vi "Login副本.vi"() -> ()   [LabVIEW 2015]
uses:
  <userlib>/QMH/Message Queue/Support/Enqueue Message (Single).vi
  <userlib>/QMH/Message Queue/Support/Enqueue Message (Array).vi
  <vilib>/Utility/error.llb/Error Cluster From Error Code.vi
  <vilib>/ErrorRing/Error Ring.xnode
  <userlib>/QMH/User Event - Stop/User Event - Stop.lvlib
  <userlib>/QMH/Message Queue/Message Queue.lvlib
panel:
  in  "Exit":bool
  in  "PassWord":string
  in  "用户名":string
  in  "Authority":u16(ring) items=["学生", "老师"]
  in  "HostThread":variant
  in  "Login":bool
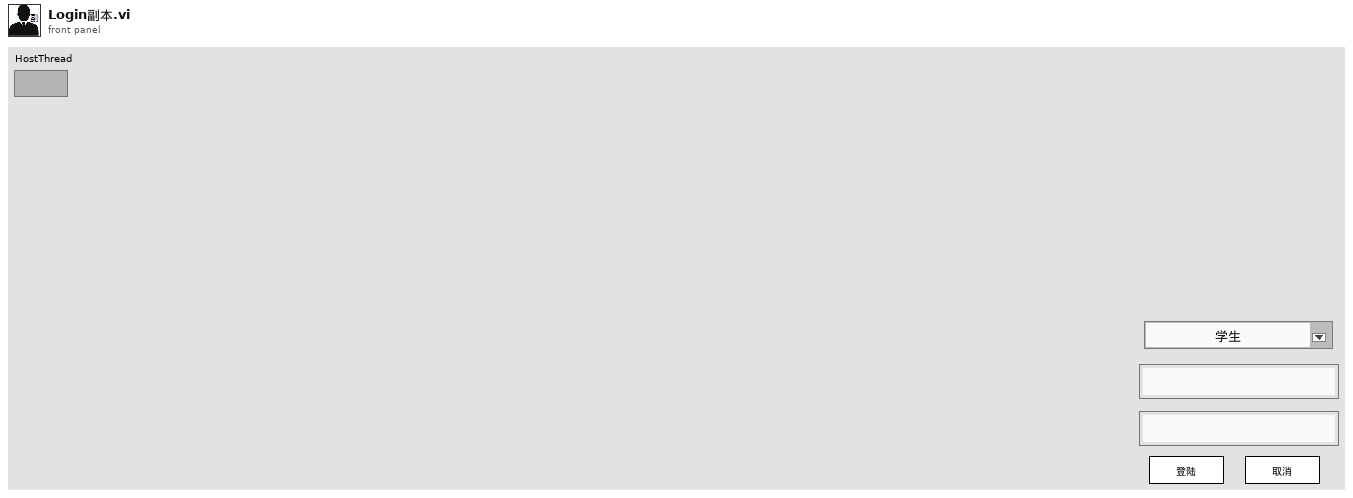
[diagram p1: front panel]
types:
  T1 = cluster{"Controls":cluster{"Exit":refnum<vi>, "Authority":refnum<vi>, "用户名":refnum<vi>, "密码":refnum<vi>}, "Thread":cluster{"ThisQ":string, "ThisVI":refnum<vi>, "HostQ":string, "HostRef":refnum<vi>, "SlavesQ":string[], "SlavesRef":refnum<vi>[]}, "Data":cluster{"Replace":bool}, "User":cluster{"Name":string}, "result?":bool}
  T2 = cluster{"用户名":refnum<vi>, "密码":refnum<vi>, "Authority":refnum<vi>}
  T3 = typedef "eventvkey.ctl" = enum16{"ASCII", "Enter", "Return", "Shift", "Ctrl", "Alt", "Cmd", "Opt", "Caps", "NumLock", "Clear", "Break", "Up", "Down", "Left", "Right", "Insert", "Delete", "Home", "End", "PageUp", "PageDown", "Escape", "Help", "Pause", "ScrollLock", "F1", "F2", "F3", "F4", "F5", "F6", "F7", "F8", "F9", "F10", "F11", "F12", "F13", "F14", "F15", "F16", "F17", "F18", "F19", "F20", "F21", "F22", "F23", "F24", "Play", "VolumeUp", "VolumeDown", "Mute", "Two Byte Char"}
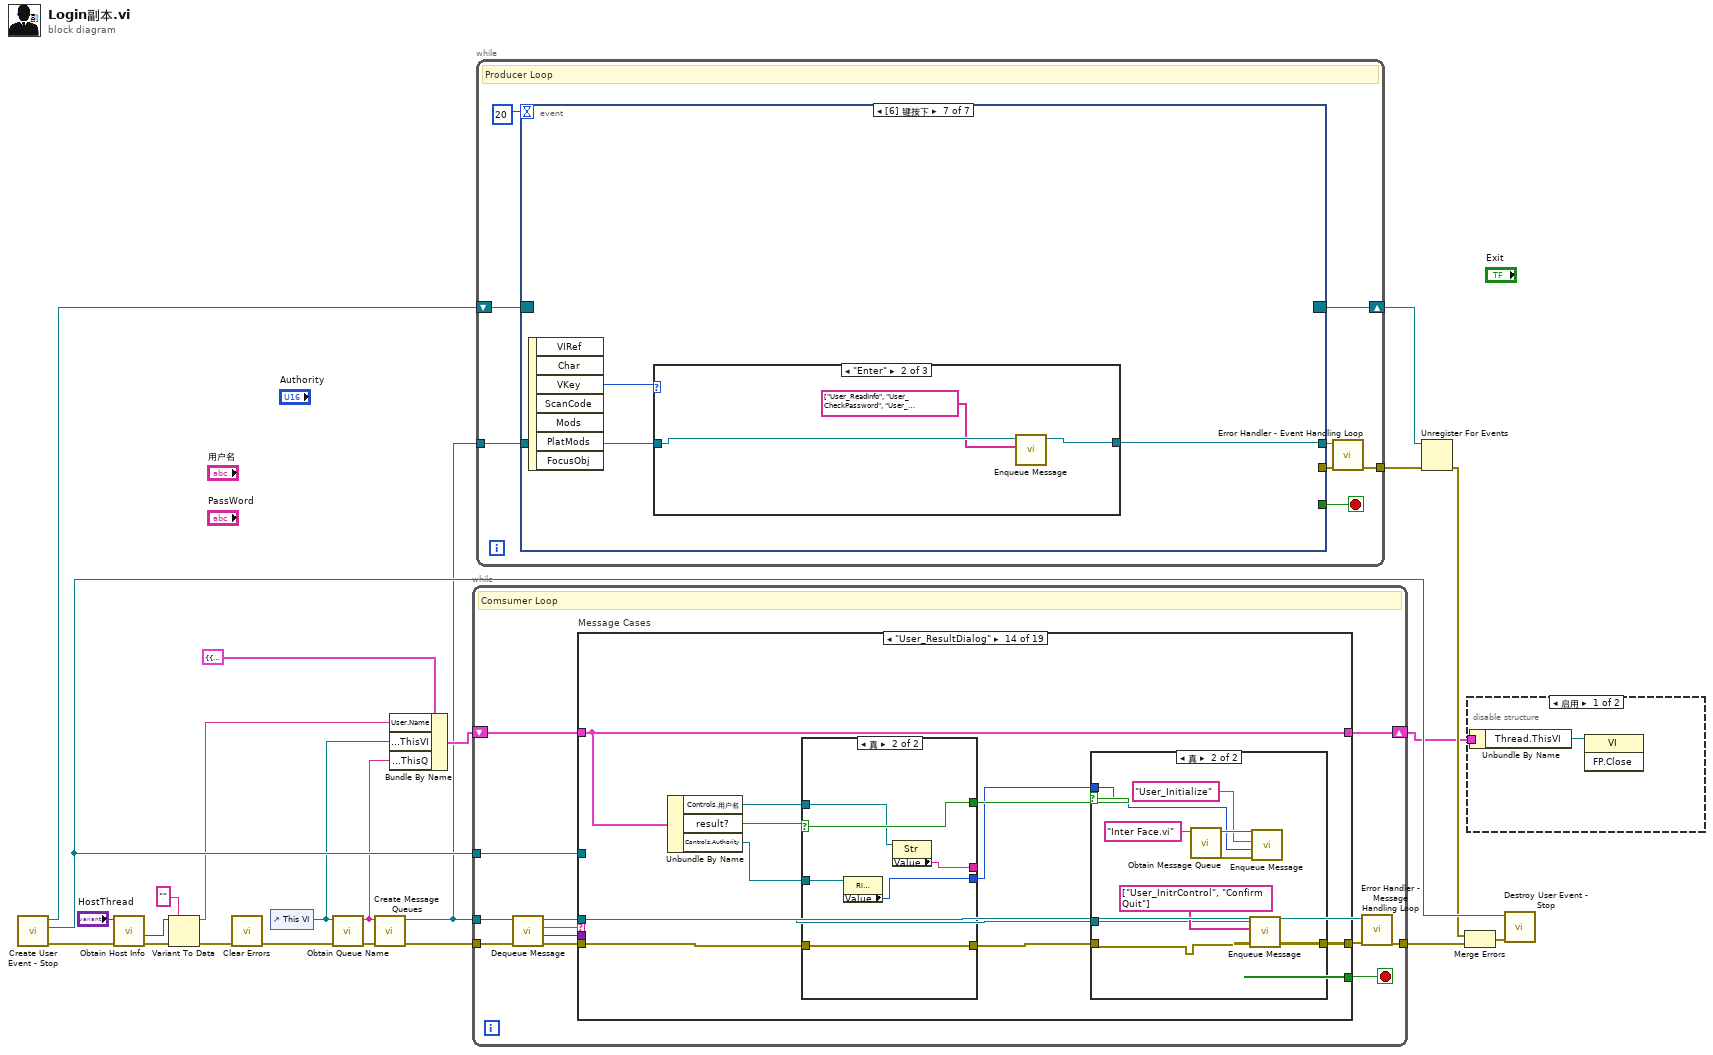
[diagram p0: block diagram]
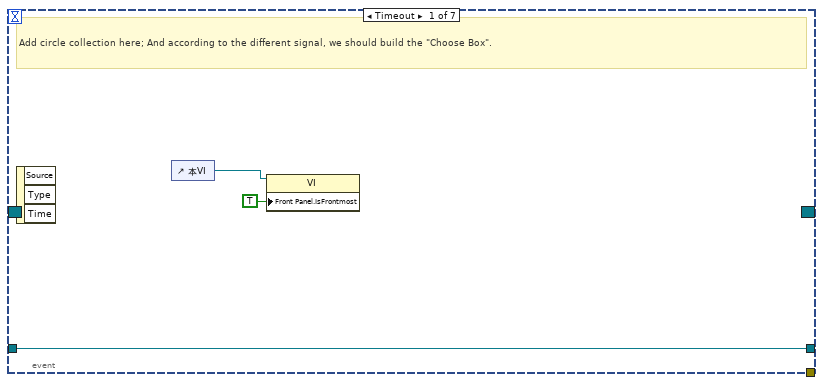
[diagram p3: hidden frame]
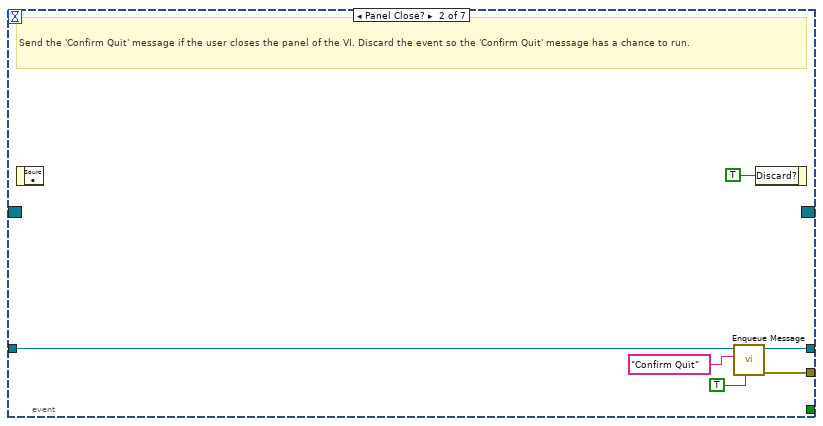
[diagram p4: hidden frame]
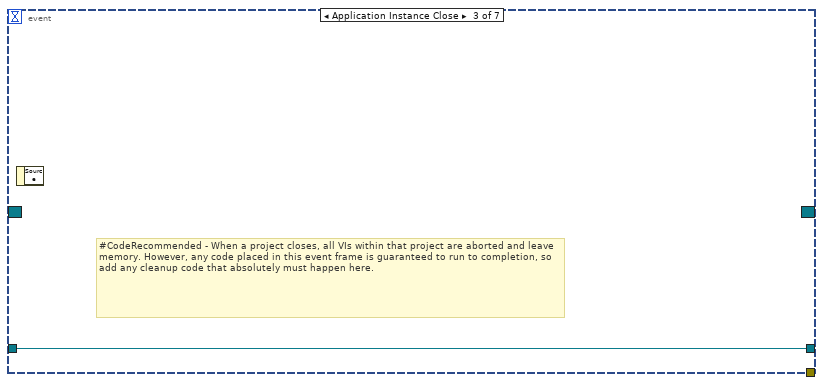
[diagram p5: hidden frame]
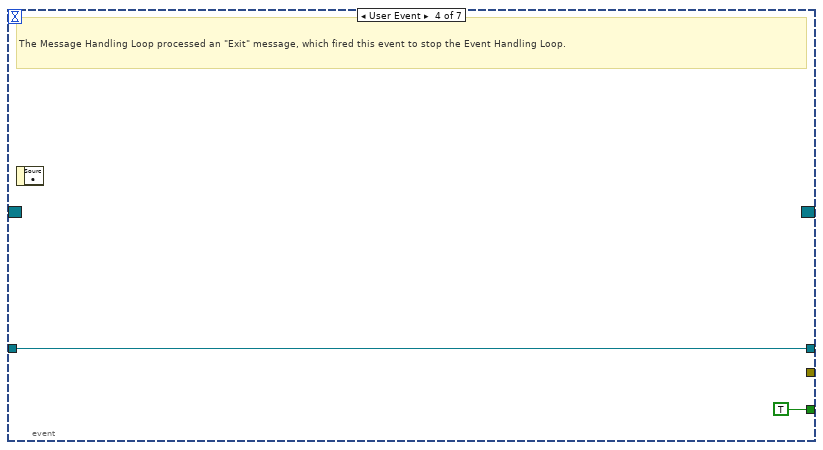
[diagram p6: hidden frame]
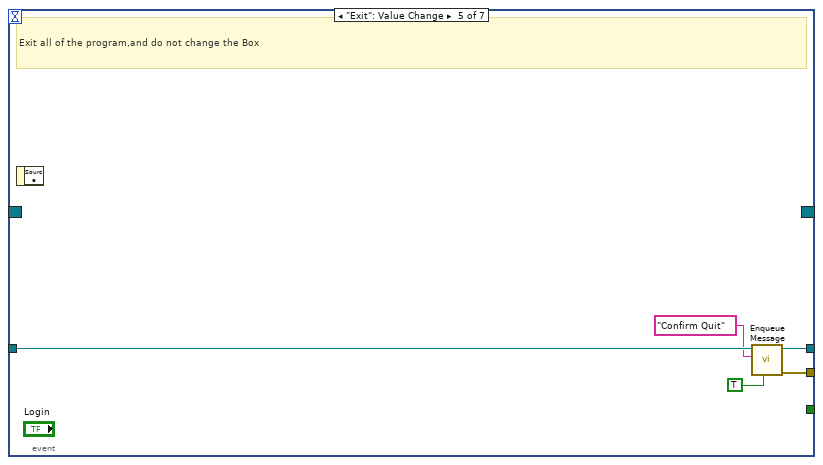
[diagram p7: hidden frame]
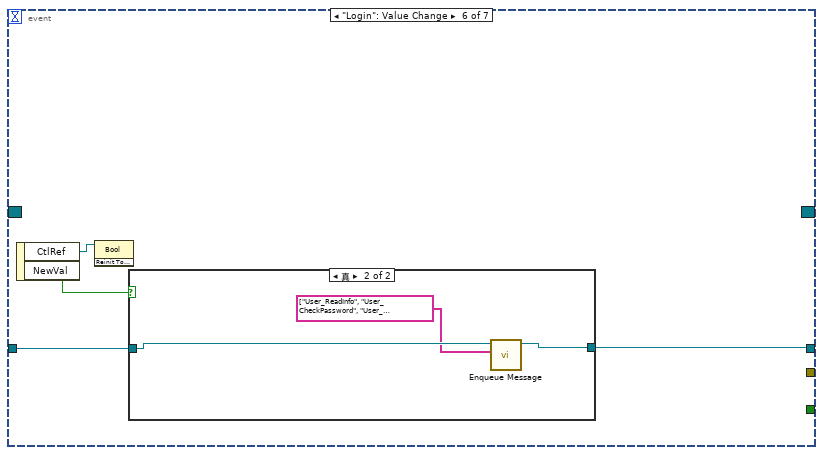
[diagram p8: hidden frame]
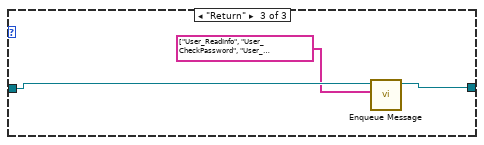
[diagram p11: hidden frame]
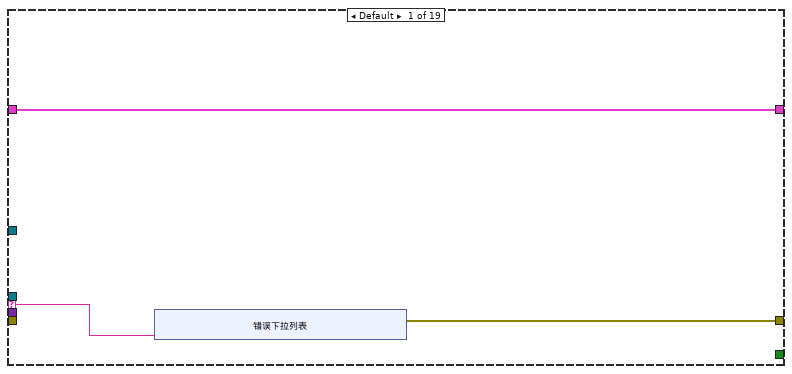
[diagram p12: hidden frame]
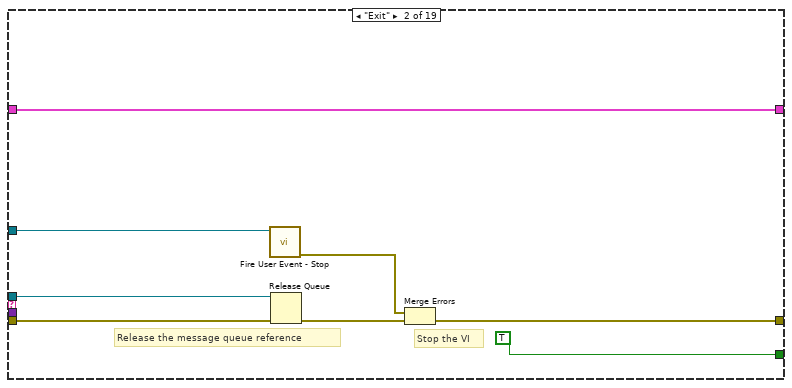
[diagram p13: hidden frame]
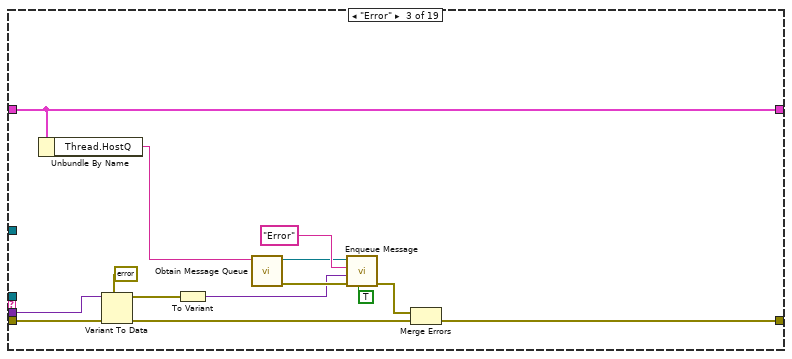
[diagram p14: hidden frame]
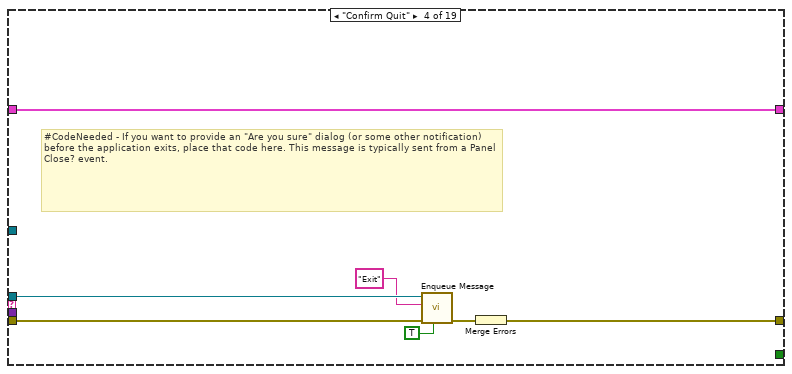
[diagram p15: hidden frame]
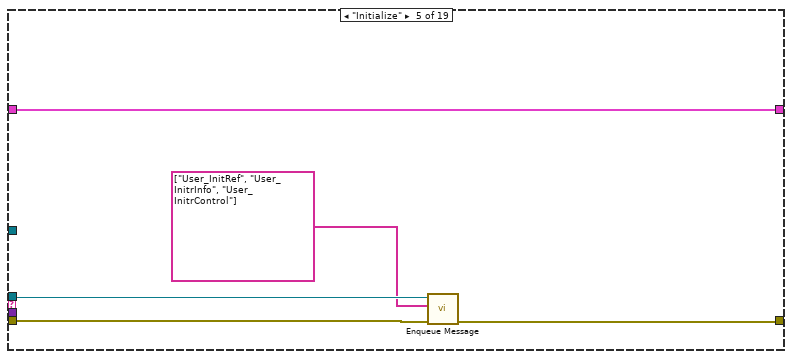
[diagram p16: hidden frame]
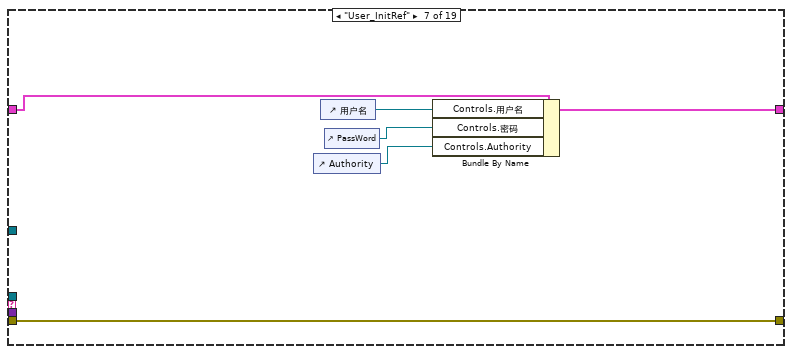
[diagram p18: hidden frame]
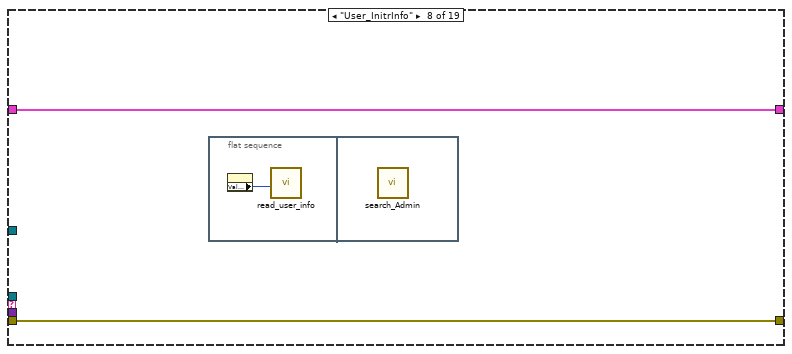
[diagram p19: hidden frame]
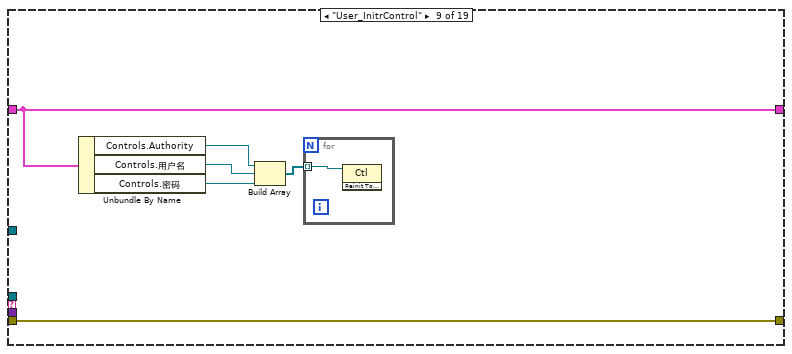
[diagram p20: hidden frame]
diagram:
  n1 = call <userlib>:"Create User Event - Stop.vi"() -> ("error out"=w10:errorcluster, "User Event - Stop"=w19:refnum<user-event>, "Stop Event Registration Refnum"=w21:refnum<event-registration>)  [unwired: 9 in]
  n2 = call <userlib>:"Obtain Host Info.vi"("error in (no error)"=w10, "HostThread"="HostThread") -> ("error out"=w7:errorcluster, "Data"=w6:variant)  [unwired: 6 in, 2 out]
  n3 = Variant To Data(error in=w7, type="", Variant=w6) -> (data=w2:string, error out=w4:errorcluster)
  n4 = call <vilib>:"Clear Errors.vi"("error in (no error)"=w4) -> ("error out"=w3:errorcluster)  [unwired: 5 in, 1 out]
  n5 = control-ref of="This VI"() -> (w12:refnum<vi>)
  n6 = call <userlib>:"Obtain Queue Name.vi"("error in (no error)"=w3, "VI Refnum"=w12) -> ("error out"=w15:errorcluster, "ViName"=w11:string)  [unwired: 8 in]
  n7 = call <userlib>:"Create Message Queues.vi"("error in (no error)"=w15, "name (unnamed)"=w11) -> ("error out"=w23:errorcluster, "QueueHandler"=w8:refnum<queue>)  [unwired: 8 in]
  n8 = Bundle By Name(cluster=T1 {"Controls"={"Exit"=refnum, "Authority"=refnum, "用户名"=refnum, "密码"=refnum}, "Thread"={"ThisQ"="", "ThisVI"=refnum, "HostQ"="", "HostRef"=refnum, "SlavesQ"=[], "SlavesRef"=[]}, "Data"={"Replace"=FALSE}, "User"={"Name"=""}, "result?"=FALSE} ("Data Cluster"), "User.Name"=w2, "Thread.ThisVI"=w12, "Thread.ThisQ"=w11) -> (w13:T1)
  n9 = while {
    tunnel: w8 -> [w27]
    shift-right: [w34] -> w1
    shift-left: w13 -> [w35]
    tunnel: w19 -> [w32]
    tunnel: w23 -> [w31]
    tunnel: [w25] -> w22
    stop <- w33 stop-if-true
    # "Comsumer Loop"
    n10 = call <userlib>:"Dequeue Message.vi"("error in (no error)"=w31, "Message Queue"=w27) -> ("error out"=w30:errorcluster, "Message Data"=w28:variant, "Message"=w29:string, "dup Message Queue"=w26:refnum<queue>)  [unwired: 6 in]
    n11 = case "Message Cases" shown="\"User_ResultDialog\"" w29 {
      selector: w29 -> [w36 _ _ _ _ _ _ _ _ _ _ _ _ _ _ _ _ _ _]
      tunnel: w26 -> [_ w53 _ w70 w76 _ _ _ _ _ _ _ _ w125 _ _ _ _ _]
      tunnel: w30 -> [_ w49 w67 w74 w78 w81 w87 w89 w96 w109 w117 w119 w121 w129 w153 w155 w157 w158 w161]
      tunnel: [w37 w50 w62 w72 w77 w81 w87 w89 w96 w109 w117 w119 w121 w127 w153 w155 w157 w158 w161] -> w24
      tunnel: w35 -> [w38 w46 w59 w73 w79 w80 w86 w88 w95 w108 w112 w118 w120 w131 w152 w154 w156 w159 w160]
      tunnel: [w38 w46 w59 w73 w79 w80 w85 w88 w95 w107 w111 w118 w120 w131 w152 w154 w156 w159 w160] -> w34
      tunnel: [_ TRUE _ _ _ _ _ _ _ _ _ _ _ _ _ _ _ _ _] -> w33
      tunnel: w28 -> [_ _ w66 _ _ _ _ _ _ _ _ _ _ _ _ _ _ _ _]
      tunnel: w32 -> [_ w48 _ _ _ _ _ _ _ _ _ _ _ _ _ _ _ _ _]
      frame Default {
        # "'Default' case only runs if there is a message that isn't defined in any of the other cases.  Output a programming error."
        n12 = xnode "错误下拉列表"("参数 0"=w36) -> ("错误输出"=w37:errorcluster)
      }
      frame "Exit" {
        # "Stop the VI"
        # "Release the message queue reference"
        # "Exit - Exit the application."
        n13 = call <userlib>:"Fire User Event - Stop.vi"("User Event - Stop"=w48) -> ("error out"=w47:errorcluster)  [unwired: 10 in]
        n14 = Release Queue(queue=w53, error in (no error)=w49) -> (error out=w51:errorcluster)  [unwired: 1 in, 2 out]
        n15 = Merge Errors(w47, w51) -> (w50:errorcluster)
      }
      frame "Error" {
        # "Error - Check the error message data and respond accordingly. This message is sent by the \"Error Handler\" VIs at the end of each loop in this application."
        n16 = Unbundle By Name(w59) -> ("Thread.HostQ"=w58:string)
        n17 = Variant To Data(error in=w67, type=errorcluster {"status"=FALSE, "code"=0, "source"=""} ("error constant"), Variant=w66) -> (data=w55:errorcluster, error out=w64:errorcluster)
        n18 = To Variant(anything=w55) -> (Variant=w54:variant)
        n19 = call <userlib>:"Obtain Message Queue.vi"("name (unnamed)"=w58) -> ("error out"=w57:errorcluster, "Message Queue"=w56:refnum<queue>)  [unwired: 9 in]
        n20 = call-poly <userlib>:"Enqueue Message.vi"("Priority Message? (F)"=TRUE, "error in (no error)"=w57, "Message Data"=w54, "Message"="Error", "Message Queue"=w56) -> ("error out"=w63:errorcluster)  [unwired: 5 in, 1 out]
        n21 = Merge Errors(w63, w64) -> (w62:errorcluster)
      }
      frame "Confirm Quit" {
        # "#CodeNeeded - If you want to provide an \"Are you sure\" dialog (or some other notification) before the application exits, place that code here. This message is typically sent from a Panel Close? event."
        # "Confirm Quit - Message that can confirm whether or not the user wants to exit the application."
        n22 = call-poly <userlib>:"Enqueue Message.vi"("Priority Message? (F)"=TRUE, "error in (no error)"=w74, "Message"="Exit", "Message Queue"=w70) -> ("error out"=w71:errorcluster)  [unwired: 6 in, 1 out]
        n23 = Merge Errors(w71) -> (w72:errorcluster)
      }
      frame "Initialize" {
        # "Initialize - Send separate messages to initialize the data and the front panel.  Bundle control references."
        n24 = call-poly <userlib>:"Enqueue Message.vi"("error in (no error)"=w78, "Message Array"=string[] ["User_InitRef", "User_InitrInfo", "User_InitrControl"], "Message Queue"=w76) -> ("error out"=w77:errorcluster)  [unwired: 7 in, 1 out]
      }
      frame "<------User------->" {
      }
      frame "User_InitRef" {
        n25 = control-ref of="Authority"() -> (w84:refnum<vi>)
        n26 = control-ref of="用户名"() -> (w83:refnum<vi>)
        n27 = control-ref of="PassWord"() -> (w82:refnum<vi>)
        n28 = Bundle By Name(cluster=w86, "Controls.用户名"=w83, "Controls.密码"=w82, "Controls.Authority"=w84) -> (w85:T1)
      }
      frame "User_InitrInfo" {
        n29 = flat-sequence {
          frame #0 {
            n30 = property on="Authority" class="Ring (严格)"() -> ("Value"=w90:u16)  [unwired: 2 in, 2 out]
            n31 = call "read_user_info.vi"("Authority"=w90) -> ()
          }
          frame #1 {
            n32 = call "search_Admin.vi"() -> ()  [unwired: 12 in]
          }
        }
      }
      frame "User_InitrControl" {
        n33 = Unbundle By Name(w95) -> ("Controls.Authority"=w94:refnum<vi>, "Controls.用户名"=w93:refnum<vi>, "Controls.密码"=w92:refnum<vi>)
        n34 = Build Array(w94, w93, w92) -> (w91:refnum<vi>[])
        n35 = for {
          tunnel: w91 -> [w97] mode=indexing
          n36 = invoke class="Ctl" method="Reinit To Default"(reference=w97) -> ()  [unwired: 2 in, 3 out]
        }
      }
      frame "User_ReadInfo" {
        n37 = Unbundle By Name(w108) -> ("Controls.用户名"=w103:refnum<vi>, "Controls.密码"=w102:refnum<vi>, "Controls.Authority"=w101:refnum<vi>)
        n38 = property on="用户名" class="Str"() -> ("Value"=w99:string)  [unwired: 2 in, 2 out]
        n39 = property on="PassWord" class="Str"() -> ("Value"=w98:string)  [unwired: 2 in, 2 out]
        n40 = property on="Authority" class="Ring (严格)"() -> ("Value"=w100:u16)  [unwired: 2 in, 2 out]
        n41 = property class="Str"(reference=w103, "Value"=w99) -> (reference out=w106:refnum<vi>)  [unwired: 1 in, 1 out]
        n42 = property class="Str"(reference=w102, "Value"=w98) -> (reference out=w105:refnum<vi>)  [unwired: 1 in, 1 out]
        n43 = property class="Ring (严格)"(reference=w101, "Value"=w100) -> (reference out=w104:refnum<vi>)  [unwired: 1 in, 1 out]
        n44 = Bundle By Name(cluster=w108, "Controls.用户名"=w106, "Controls.密码"=w105, "Controls.Authority"=w104) -> (w107:T1)
      }
      frame "User_CheckPassword" {
        n45 = Unbundle By Name(w112) -> ("Controls.用户名"=w116:refnum<vi>, "Controls.密码"=w115:refnum<vi>, "Controls.Authority"=w114:refnum<vi>)
        n46 = Bundle("用户名"=w116, "密码"=w115, "Authority"=w114) -> (w113:T2)  [unwired: 1 in]
        n47 = call "check_password.vi"("Ref"=w113) -> ("result？"=w110:bool)
        n48 = Bundle By Name(cluster=w112, "result?"=w110) -> (w111:T1)
      }
      frame "User_Add" {
      }
      frame "User_Delete" {
      }
      frame "User_ResultDialog" {
        n49 = Unbundle By Name(w131) -> ("Controls.用户名"=w124:refnum<vi>, "result?"=w130:bool, "Controls.Authority"=w122:refnum<vi>)
        n50 = case shown="真" w130 {
          selector: w130 -> [w144 w151]
          tunnel: [_ w146] -> w123
          tunnel: w129 -> [w145 w150]
          tunnel: [w145 w150] -> w126
          tunnel: [w144 w151] -> w128
          tunnel: w124 -> [_ w149]
          tunnel: ["未登陆用户" ("Value") w148] -> _
          tunnel: w122 -> [_ w147]
          frame False {
            n51 = One Button Dialog(message="用户名或密码错误！" ("Message")) -> ()  [unwired: 1 in, 1 out]
          }
          frame True {
            n52 = property class="Ring (严格)"(reference=w147) -> ("Value"=w146:u16)  [unwired: 1 in, 2 out]
            n53 = property class="Str"(reference=w149) -> ("Value"=w148:string)  [unwired: 1 in, 2 out]
          }
        }
        n54 = case shown="真" w128 {
          tunnel: [w132 w138] -> w127
          tunnel: w126 -> [w132 w139]
          tunnel: w125 -> [_ w140]
          tunnel: w123 -> [_ w133]
          frame False {
          }
          frame True {
            n55 = call <userlib>:"Obtain Message Queue.vi"("name (unnamed)"="Inter Face.vi") -> ("error out"=w134:errorcluster, "Message Queue"=w137:refnum<queue>)  [unwired: 9 in]
            n56 = call-poly <userlib>:"Enqueue Message.vi"("error in (no error)"=w139, "Message Array"=string[] ["User_InitrControl", "Confirm Quit"], "Message Queue"=w140) -> ("error out"=w138:errorcluster)  [unwired: 7 in, 1 out]
            n57 = call-poly <userlib>:"Enqueue Message.vi"("error in (no error)"=w134, "Message Data"=w133, "Message"="User_Initialize", "Message Queue"=w137) -> ()  [unwired: 6 in, 2 out]
          }
        }
      }
      frame "<-------UI-------->" {
      }
      frame "Init_controls" {
      }
      frame "<------Core------>" {
      }
      frame "Core_InitializeRef" {
        # "Initialize control references. For there is not enough space to locate all the control references, separate the codes into 2 messages"
      }
      frame "<---Operation--->" {
      }
    }
    n58 = call <userlib>:"Error Handler - Message Handling Loop.vi"("error in (no error)"=w24, "Message Queue"=w26) -> ("dup error in"=w25:errorcluster)  [unwired: 8 in, 1 out]
  }
  n59 = while {
    tunnel: w8 -> [w169]
    shift-right: [w167] -> w17
    shift-left: w21 -> [w168]
    tunnel: [w163] -> w16
    stop <- w165 stop-if-true
    # "Producer Loop"
    n60 = event shown="[6] 键按下" {
      selector: w168 -> [_ _ _ _ _ _ _]
      dyn-events: [_ _ _ _ _ _ _] -> w167
      timeout: 20 -> [_ _ _ _ _ _ _]
      tunnel: [_ _ _ TRUE ("Discard?") _ _ _] -> w165
      tunnel: w169 -> [w172 w177 w179 w181 w186 w190 w197]
      tunnel: [_ w176 _ _ w184 _ _] -> w166
      tunnel: [w172 w175 w179 w181 w185 w189 w196] -> w164
      event Timeout {
        # "Add circle collection here; And according to the different signal, we should build the \"Choose Box\"."
        n61 = event-data() -> ()  [unwired: 1 in, 3 out]
        n62 = control-ref of="本VI"() -> (w170:refnum<vi>)
        n63 = property class="VI"(reference=w170, "Front Panel.IsFrontmost"=TRUE ("前面板窗口:在最前")) -> ()  [unwired: 1 in, 2 out]
      }
      event Panel Close? {
        # "Send the 'Confirm Quit' message if the user closes the panel of the VI. Discard the event so the 'Confirm Quit' message has a chance to run."
        n64 = event-data() -> ()  [unwired: 1 in, 1 out]
        n65 = call-poly <userlib>:"Enqueue Message.vi"("Priority Message? (F)"=TRUE, "Message"="Confirm Quit", "Message Queue"=w177) -> ("error out"=w176:errorcluster, "dup Message Queue"=w175:refnum<queue>)  [unwired: 7 in]
        n66 = event-data("Discard?"=TRUE) -> ()  [unwired: 1 in, 1 out]
      }
      event Application Instance Close {
        # "#CodeRecommended - When a project closes, all VIs within that project are aborted and leave memory. However, any code placed in this event frame is guaranteed to run to completion, so add any cleanup code that absolutely must happen here."
        n67 = event-data() -> ()  [unwired: 1 in, 1 out]
      }
      event User Event {
        # "The Message Handling Loop processed an \"Exit\" message, which fired this event to stop the Event Handling Loop."
        n68 = event-data() -> ()  [unwired: 1 in, 1 out]
      }
      event "Exit": Value Change {
        # "Exit all of the program,and do not change the Box"
        n69 = event-data() -> ()  [unwired: 1 in, 1 out]
        n70 = call-poly <userlib>:"Enqueue Message.vi"("Priority Message? (F)"=TRUE, "Message"="Confirm Quit", "Message Queue"=w186) -> ("error out"=w184:errorcluster, "dup Message Queue"=w185:refnum<queue>)  [unwired: 7 in]
      }
      event "Login": Value Change {
        n71 = event-data() -> ("CtlRef"=w187:refnum<vi>, "NewVal"=w188:bool)  [unwired: 1 in]
        n72 = invoke class="Bool" method="Reinit To Default"(reference=w187) -> ()  [unwired: 2 in, 3 out]
        n73 = case shown="真" w188 {
          tunnel: w190 -> [w191 w194]
          tunnel: [w191 w193] -> w189
          frame False {
          }
          frame True {
            n74 = call-poly <userlib>:"Enqueue Message.vi"("Message Array"=string[] ["User_ReadInfo", "User_CheckPassword", "User_ResultDialog"], "Message Queue"=w194) -> ("dup Message Queue"=w193:refnum<queue>)  [unwired: 8 in, 1 out]
          }
        }
      }
      event Key Down {
        n75 = event-data() -> ("VKey"=w195:T3)  [unwired: 1 in, 6 out]
        n76 = case shown="\"Enter\"" w195 {
          tunnel: w197 -> [w198 w201 w204]
          tunnel: [w198 w200 w203] -> w196
          frame "ASCII", Default {
          }
          frame "Enter" {
            n77 = call-poly <userlib>:"Enqueue Message.vi"("Message Array"=string[] ["User_ReadInfo", "User_CheckPassword", "User_ResultDialog"], "Message Queue"=w201) -> ("dup Message Queue"=w200:refnum<queue>)  [unwired: 8 in, 1 out]
          }
          frame "Return" {
            n78 = call-poly <userlib>:"Enqueue Message.vi"("Message Array"=string[] ["User_ReadInfo", "User_CheckPassword", "User_ResultDialog"], "Message Queue"=w204) -> ("dup Message Queue"=w203:refnum<queue>)  [unwired: 8 in, 1 out]
          }
        }
      }
    }
    n79 = call <userlib>:"Error Handler - Event Handling Loop.vi"("error in (no error)"=w166, "Message Queue"=w164) -> ("dup error in"=w163:errorcluster)  [unwired: 8 in, 1 out]
  }
  n80 = Unregister For Events(event registration refnum=w17, error in=w16) -> (error out=w18:errorcluster)
  n81 = Merge Errors(w18, w22) -> (w20:errorcluster)
  n82 = disable-structure shown="启用" {
    disable-tunnel: w1 -> [w206 _]
    frame Enabled {
      n83 = Unbundle By Name(w206) -> ("Thread.ThisVI"=w205:refnum<vi>)
      n84 = invoke class="VI" method="FP.Close"(reference=w205) -> ()  [unwired: 2 in, 3 out]
    }
    frame Disabled {
    }
  }
  n85 = call <userlib>:"Destroy User Event - Stop.vi"("error in (no error)"=w20, "User Event - Stop"=w19) -> ()  [unwired: 9 in, 1 out]
